vi "Step Adjust.vi"(8 "error in (no error)":errorcluster, 11 "LargeScrollbar in":refnum<class "LargeScrollbar.lvclass">) -> (0 "error out":errorcluster, 2 "Step out":i32, 3 "LargeScrollbar out":refnum<class "LargeScrollbar.lvclass">)   [LabVIEW 2015, in "LargeScrollbar.lvclass"]
doc: "<b> </b> <b> </b>\n©2016 Q Software Innovations, LLC (QSI)\nwritten by Quentin Alldredge\nproduced in LabVIEW 2015\n\nsupport@qsoftwareinnovations.com\nwww.qsoftwareinnovations.com\n\nAll rights reserved.\n\nRedistribution and use in source and binary forms, with or without modification, are permitted provided that the following conditions are met:\n\n * Redistributions of source code must retain the above copyright notice, this list of conditions and the following disclaimer.\n * Redistributions in binary form must reproduce the above copyright notice, this list of conditions and the following disclaimer in the documentation and/or other materials provided with the distribution.\n * Neither the name of Q Software Innovations, LLC. nor the names of its contributors may be used to endorse or promote products derived from this software without specific prior written permission.\n\nTHIS SOFTWARE IS PROVIDED BY THE COPYRIGHT HOLDERS AND CONTRIBUTORS \"AS IS\" AND ANY EXPRESS OR IMPLIED WARRANTIES, INCLUDING, BUT NOT LIMITED TO, THE IMPLIED WARRANTIES OF MERCHANTABILITY AND FITNESS FOR A PARTICULAR PURPOSE ARE DISCLAIMED. IN NO EVENT SHALL THE COPYRIGHT OWNER OR CONTRIBUTORS BE LIABLE FOR ANY DIRECT, INDIRECT, INCIDENTAL, SPECIAL, EXEMPLARY, OR CONSEQUENTIAL DAMAGES (INCLUDING, BUT NOT LIMITED TO, PROCUREMENT OF SUBSTITUTE GOODS OR SERVICES; LOSS OF USE, DATA, OR PROFITS; OR BUSINESS INTERRUPTION) HOWEVER CAUSED AND ON ANY THEORY OF LIABILITY, WHETHER IN CONTRACT, STRICT LIABILITY, OR TORT (INCLUDING NEGLIGENCE OR OTHERWISE) ARISING IN ANY WAY OUT OF THE USE OF THIS SOFTWARE, EVEN IF ADVISED OF THE POSSIBILITY OF SUCH DAMAGE."
uses:
  LargeScrollbar.lvclass
  LargeScrollbar.lvclass/LargeScrollbar.ctl
  Read Timeout Iteration.vi
  Write Timeout Iteration.vi
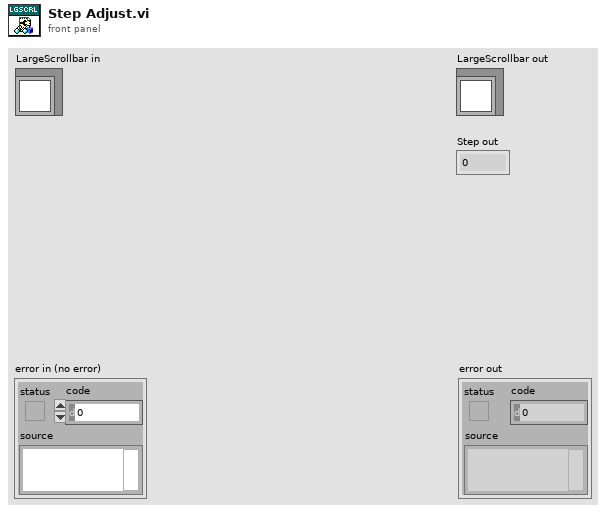
[diagram p1: front panel]
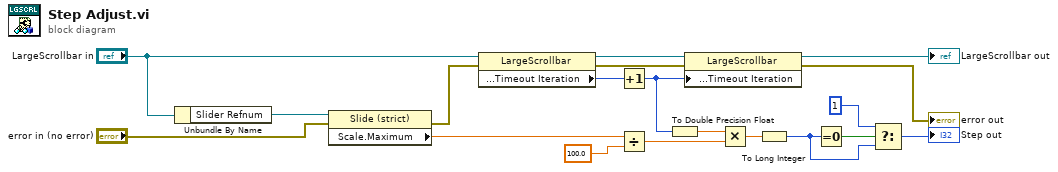
[diagram p0: block diagram]
diagram:
  n1 = Unbundle By Name("LargeScrollbar in") -> ("Slider Refnum"=w18:refnum<vi>)
  n2 = property class="Slide (strict)"(reference=w18, error in="error in (no error)") -> (error out=w3:errorcluster, "Scale.Maximum"=w17:dbl)  [unwired: 1 out]
  n3 = property class="LargeScrollbar"(reference="LargeScrollbar in", error in=w3) -> (reference out=w8:refnum<class "LargeScrollbar.lvclass">, error out=w7:errorcluster, "State Data:Accessors:Timeout Iteration"=w9:u32)
  n4 = Increment(x=w9) -> (x+1=w6:u32)
  n5 = Divide(x=w17, y=100.0) -> (x/y=w15:dbl)
  n6 = To Double Precision Float(number=w6) -> (double precision float=w16:dbl)
  n7 = property class="LargeScrollbar"(reference=w8, error in=w7, "State Data:Accessors:Timeout Iteration"=w6) -> (reference out=→"LargeScrollbar out":refnum<class "LargeScrollbar.lvclass">, error out=→"error out":errorcluster)
  n8 = Multiply(x=w16, y=w15) -> (x*y=w14:dbl)
  n9 = To Long Integer(number=w14) -> (32bit integer=w12:i32)
  n10 = Equal To 0?(x=w12) -> (x = 0?=w13:bool)
  n11 = Select(t=1, s=w13, f=w12) -> (s? t:f=→"Step out":i32)
